vi "get_version_from_git.vi"(0 "path_project":path) -> (1 "Version":string, 2 "return code":i32)   [LabVIEW 2018]
panel:
  out "standard error":string
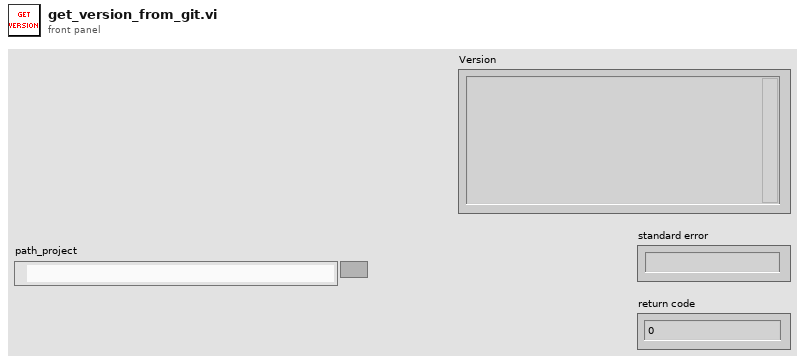
[diagram p1: front panel]
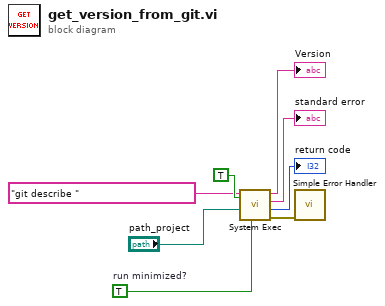
[diagram p0: block diagram]
diagram:
  w5 = TRUE  # run minimized?
  n1 = call <vilib>:"System Exec.vi"("run minimized? (F)"=w5, "wait until completion? (T)"=TRUE, "working directory"="path_project", "command line"="git describe ") -> ("error out"=w6:errorcluster, "return code"=→"return code":i32, "standard error"=→"standard error":string, "standard output"=→"Version":string)  [unwired: 2 in, 2 out]
  n2 = call <vilib>:"Simple Error Handler.vi"("error in (no error)"=w6) -> ()  [unwired: 1 in, 8 out]
